vi "Switch_RaiseEdgeEvent.vi"(6 "Old通道2":bool, 7 "Old通道1":bool, 8 "错误输入（无错误）":errorcluster, 10 "用户事件":refnum<user-event>, 11 "COM":refnum<visa-resource-name>) -> (0 "错误输出":errorcluster, 1 "通道2":bool, 2 "通道1":bool, 3 "COM Out":refnum<visa-resource-name>)   [LabVIEW 2018, in "Switch.lvlib"]
uses:
  Switch.lvlib
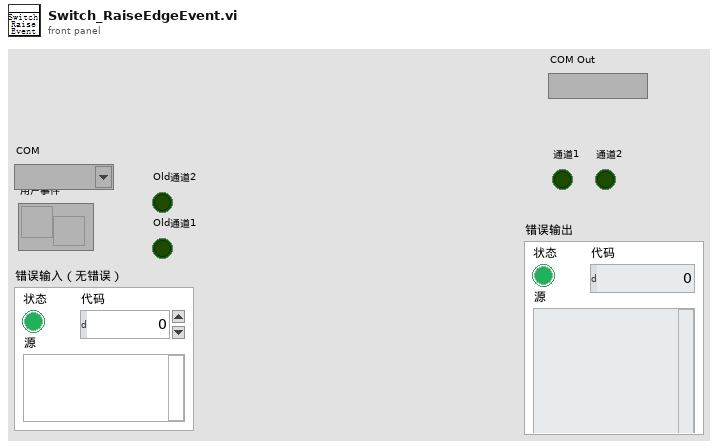
[diagram p1: front panel]
types:
  T1 = typedef "触发方式枚举.ctl" = enum16{"上升沿", "下降沿"}
  T2 = typedef "通道枚举.ctl" = enum16{"通道1", "通道2"}
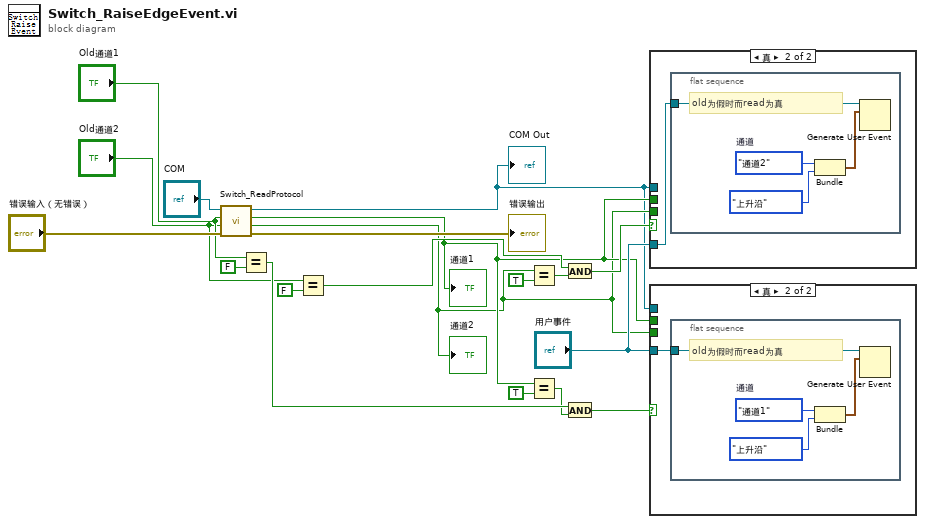
[diagram p0: block diagram]
diagram:
  n1 = call "Switch_ReadProtocol.vi"("错误输入（无错误）"="错误输入（无错误）", "Old通道2"="Old通道2", "Old通道1"="Old通道1", "COM"="COM") -> ("错误输出"=→"错误输出":errorcluster, "通道2"=w2:bool, "通道1"=w3:bool, "COM Out"=w1:refnum<visa-resource-name>)  [unwired: 4 in]
  "COM Out" <- w1
  "通道1" <- w3
  "通道2" <- w2
  n2 = Equal?(x="Old通道1", y=FALSE) -> (x = y?=w13:bool)
  n3 = Equal?(x="Old通道2", y=FALSE) -> (x = y?=w8:bool)
  n4 = Equal?(x=w2, y=TRUE) -> (x = y?=w7:bool)
  n5 = Equal?(x=w3, y=TRUE) -> (x = y?=w12:bool)
  n6 = And(x=w8, y=w7) -> (x .and. y?=w5:bool)
  n7 = And(x=w13, y=w12) -> (x .and. y?=w11:bool)
  n8 = case shown="真" w5 {
    tunnel: "用户事件" -> [_ w20]
    tunnel: w1 -> [_ _]
    tunnel: w3 -> [_ _]
    tunnel: w2 -> [_ _]
    frame False {
    }
    frame True {
      n9 = flat-sequence {
        tunnel: w20 -> [w24]
        frame #0 {
          w22 = 通道枚举."通道2"  # 通道
          # "old为假时而read为真"
          n10 = Bundle("通道"=w22, "触发方式"=触发方式枚举."上升沿") -> (w23:cluster{"通道":T2, "触发方式":T1})  [unwired: 1 in]
          n11 = Generate User Event(user event=w24, event data cluster=w23) -> ()  [unwired: 2 in, 2 out]
        }
      }
    }
  }
  n12 = case shown="真" w11 {
    tunnel: "用户事件" -> [_ w25]
    tunnel: w3 -> [_ _]
    tunnel: w2 -> [_ _]
    tunnel: w1 -> [_ _]
    frame False {
    }
    frame True {
      n13 = flat-sequence {
        tunnel: w25 -> [w29]
        frame #0 {
          w27 = 通道枚举."通道1"  # 通道
          # "old为假时而read为真"
          n14 = Bundle("通道"=w27, "触发方式"=触发方式枚举."上升沿") -> (w28:cluster{"通道":T2, "触发方式":T1})  [unwired: 1 in]
          n15 = Generate User Event(user event=w29, event data cluster=w28) -> ()  [unwired: 2 in, 2 out]
        }
      }
    }
  }
